vi "compute_zernike_coeffs.vi"() -> ()   [LabVIEW 2020]
uses:
  ComputePhaseSet.lvclass
  HasoSlopes.lvclass
  Pupil.lvclass
  CircularPupilDetectionParams.ctl
  PupilDetectionOption.ctl
  CircularAutoDetectionOptions.ctl
  PupilDetectionMode.ctl
  ZernikeModalPrefs.ctl
  ZernikeProjectionPupilSetup.ctl
  Point2Df.ctl
  ModalCoef.lvclass
  HasoData.lvclass
  WavefrontReconstructionMode.ctl
  WavefrontModalReconstructionType.ctl
panel:
  out "Zernike pupil":i32[][](graph)
  out "Zernike Coefficients":sgl[](graph)
  in  "Haso slopes file name":string="Data\\data_phase_computation.has"
  out "error out":errorcluster
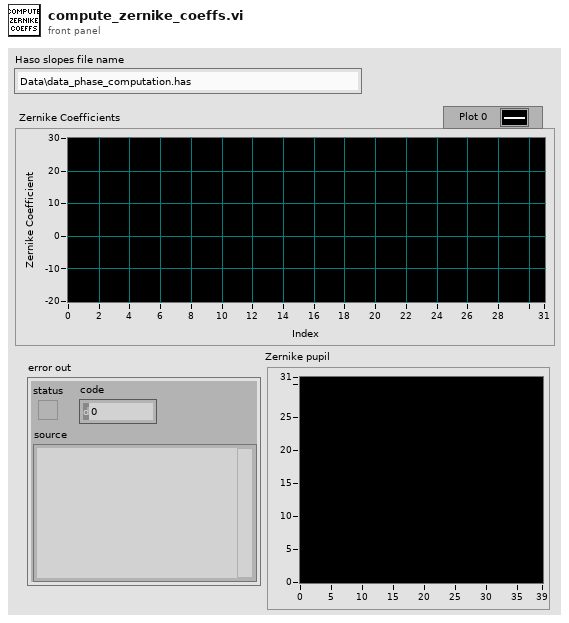
[diagram p1: front panel]
types:
  T1 = typedef "WavefrontModalReconstructionType.ctl" = enum16{"Legendre", "Zernike"}
  T2 = typedef "WavefrontReconstructionMode.ctl" = enum16{"None", "Modal_Legendre", "Modal_Zernike", "Zonal", "Modal_Zonal_Zernike", "Modal_Zonal_Legendre"}
  T3 = typedef "ZernikeModalPrefs.ctl" = cluster{"Number of coefficients":u32, "Filtered coefficients":u32[], "RMS Zernike normalization":bool, "CircularProjectionPupilDimensions":T4}
  T4 = typedef "ZernikeProjectionPupilSetup.ctl" = cluster{"Pupil center_sspp":T5, "Pupil radius_sspp":sgl}
  T5 = typedef "Point2Df.ctl" = cluster{"X":sgl, "Y":sgl}
  T6 = typedef "CircularPupilDetectionParams.ctl" = cluster{"PupilDetectionOption":T7, "AutoDetectionOption":T8, "PupilDetectionMode":T9, "CentralOccultationDetection":bool}
  T7 = typedef "PupilDetectionOption.ctl" = enum16{"Manual", "Automatic"}
  T8 = typedef "CircularAutoDetectionOptions.ctl" = enum16{"manual_radius_auto_center", "manual_center_auto_radius", "auto_radius_auto_center"}
  T9 = typedef "PupilDetectionMode.ctl" = enum16{"inscribed", "circumscribed"}
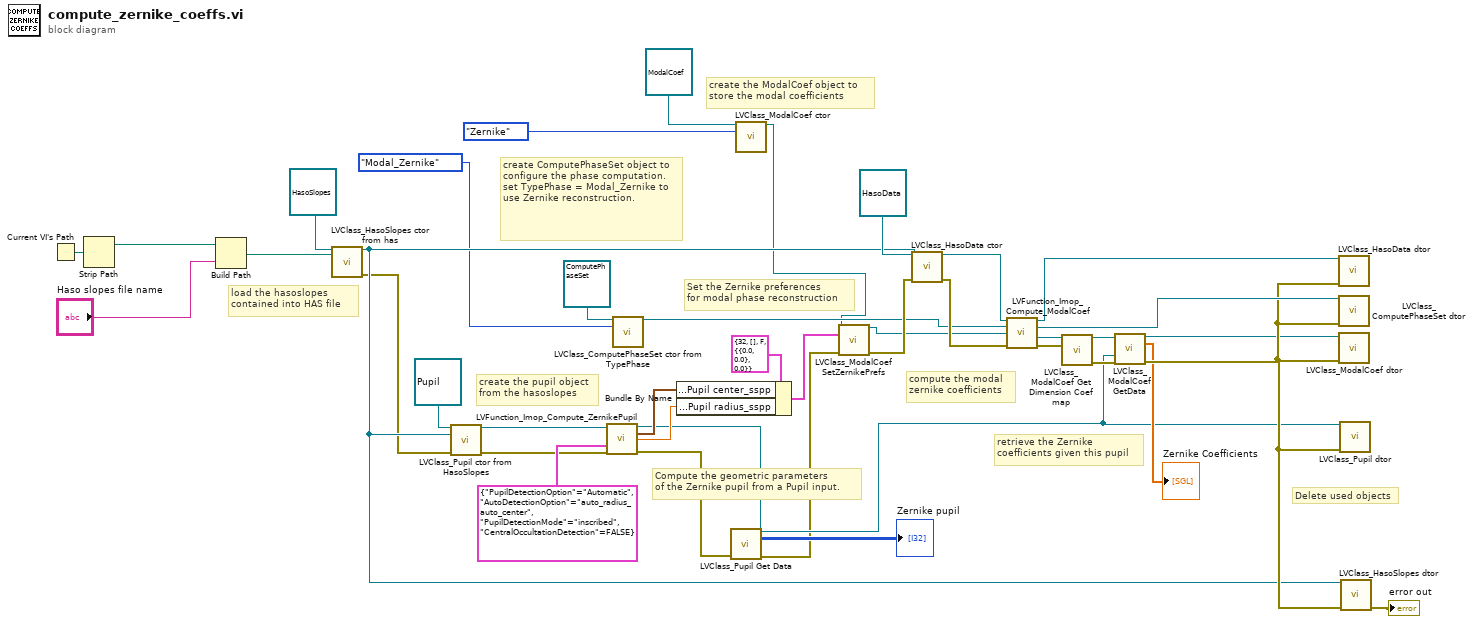
[diagram p0: block diagram]
diagram:
  # "Delete used objects"
  # "retrieve the Zernike\ncoefficients given this pupil"
  # "compute the modal\nzernike coefficients"
  # "create the ModalCoef object to\nstore the modal coefficients"
  # "Set the Zernike preferences\nfor modal phase reconstruction"
  # "Compute the geometric parameters\nof the Zernike pupil from a Pupil input."
  # "create the pupil object\nfrom the hasoslopes"
  # "load the hasoslopes\ncontained into HAS file"
  # "create ComputePhaseSet object to configure the phase computation.\nset TypePhase = Modal_Zernike to use Zernike reconstruction."
  n1 = Current VI's Path() -> (path=w16:path)
  n2 = Strip Path(path=w16) -> (stripped path=w13:path)  [unwired: 1 out]
  n3 = Build Path(base path=w13, name or relative path="Haso slopes file name") -> (appended path=w14:path)
  n4 = call "LVClass_HasoSlopes ctor from has.vi"("HasoSlopes (const)"=refnum<class "HasoSlopes.lvclass"> refnum ("HasoSlopes in"), ".has path"=w14) -> ("HasoSlopes (new)"=w26:refnum<class "HasoSlopes.lvclass">, "error out"=w12:errorcluster)  [unwired: 12 in]
  n5 = call "LVClass_Pupil ctor from HasoSlopes.vi"("Pupil (const)"=refnum<class "Pupil.lvclass"> refnum ("Pupil in"), "HasoSlopes"=w26, "error in (no error)"=w12) -> ("Pupil (new)"=w38:refnum<class "Pupil.lvclass">, "error out"=w36:errorcluster)  [unwired: 10 in, 1 out]
  n6 = call "LVFunction_Imop_Compute_ZernikePupil.vi"("Pupil.lvclass"=w38, "CircularPupilDetectionParams"=T6 {"PupilDetectionOption"=enum."Automatic", "AutoDetectionOption"=enum."auto_radius_auto_center", "PupilDetectionMode"=enum."inscribed", "CentralOccultationDetection"=FALSE}, "error in"=w36) -> ("Pupil.lvclass"=w8:refnum<class "Pupil.lvclass">, "center"=w18:T5, "radius"=w17:sgl, "error out"=w6:errorcluster)  [unwired: 9 in]
  n7 = call "LVClass_ComputePhaseSet ctor from TypePhase.vi"("ComputePhaseSet (const)"=refnum<class "ComputePhaseSet.lvclass"> refnum ("ComputePhaseSet in"), "TypePhase"=WavefrontReconstructionMode."Modal_Zernike") -> ("ComputePhaseSet (new)"=w3:refnum<class "ComputePhaseSet.lvclass">)  [unwired: 12 in, 1 out]
  n8 = Bundle By Name(cluster=T3 {"Number of coefficients"=32, "Filtered coefficients"=[], "RMS Zernike normalization"=FALSE, "CircularProjectionPupilDimensions"={"Pupil center_sspp"={"X"=0.0, "Y"=0.0}, "Pupil radius_sspp"=0.0}} ("ZernikeModalPrefs"), "CircularProjectionPupilDimensions.Pupil center_sspp"=w18, "CircularProjectionPupilDimensions.Pupil radius_sspp"=w17) -> (w19:T3)
  n9 = call "LVClass_Pupil Get Data.vi"("Pupil in"=w8, "error in (no error)"=w6) -> ("Pupil out"=w7:refnum<class "Pupil.lvclass">, "Data"=→"Zernike pupil":i32[][], "error out"=w5:errorcluster)  [unwired: 11 in]
  n10 = call "LVClass_ModalCoef ctor.vi"("ModalCoef (const)"=refnum<class "ModalCoef.lvclass"> refnum ("ModalCoef in"), "TypePhase"=WavefrontModalReconstructionType."Zernike") -> ("ModalCoef (new)"=w1:refnum<class "ModalCoef.lvclass">)  [unwired: 12 in, 1 out]
  n11 = call "LVClass_ModalCoef SetZernikePrefs.vi"("ModalCoef in"=w1, "ZernikeModalPrefs"=w19, "error in (no error)"=w5) -> ("ModalCoef out"=w2:refnum<class "ModalCoef.lvclass">, "error out"=w22:errorcluster)  [unwired: 11 in]
  n12 = call "LVClass_HasoData ctor.vi"("HasoData (const)"=refnum<class "HasoData.lvclass"> refnum ("HasoData in"), "HasoSlopes"=w26, "error in (no error)"=w22) -> ("HasoData (new)"=w33:refnum<class "HasoData.lvclass">, "error out"=w23:errorcluster)  [unwired: 10 in, 1 out]
  n13 = call "LVFunction_Imop_Compute_ModalCoef.vi"("HasoData.lvclass"=w33, "ComputePhaseSet.lvclass"=w3, "ModalCoef.lvclass"=w2, "error constant"=w23) -> ("HasoData.lvclass (dup)"=w28:refnum<class "HasoData.lvclass">, "ComputePhaseSet.lvclass (dup)"=w30:refnum<class "ComputePhaseSet.lvclass">, "ModalCoef.lvclass (dup)"=w32:refnum<class "ModalCoef.lvclass">, "error out"=w24:errorcluster)  [unwired: 8 in]
  n14 = call "LVClass_ModalCoef Get Dimension Coef map.vi"("ModalCoef in"=w32, "error in (no error)"=w24) -> ("ModalCoef out"=w31:refnum<class "ModalCoef.lvclass">, "error out"=w25:errorcluster)  [unwired: 11 in, 1 out]
  n15 = call "LVClass_ModalCoef GetData.vi"("ModalCoef in"=w31, "Pupil.lvclass"=w7, "error in (no error)"=w25) -> ("ModalCoef out"=w27:refnum<class "ModalCoef.lvclass">, "coef"=→"Zernike Coefficients":sgl[], "error out"=w29:errorcluster)  [unwired: 8 in, 2 out]
  n16 = call "LVClass_HasoData dtor.vi"("HasoData in"=w28, "error in (no error)"=w29) -> ()  [unwired: 12 in, 2 out]
  n17 = call "LVClass_ComputePhaseSet dtor.vi"("ComputePhaseSet in"=w30, "error in (no error)"=w29) -> ()  [unwired: 12 in, 2 out]
  n18 = call "LVClass_ModalCoef dtor.vi"("ModalCoef in"=w27, "error in (no error)"=w29) -> ()  [unwired: 12 in, 2 out]
  n19 = call "LVClass_Pupil dtor.vi"("Pupil in"=w7, "error in (no error)"=w29) -> ()  [unwired: 12 in, 2 out]
  n20 = call "LVClass_HasoSlopes dtor.vi"("HasoSlopes in"=w26, "error in (no error)"=w29) -> ("error out"=→"error out":errorcluster)  [unwired: 12 in, 1 out]
